vi "MATglobal.vi"(1 "s":bool, 2 "rawdata":T1) -> (0 "rawdata":T1)   [LabVIEW 2009]
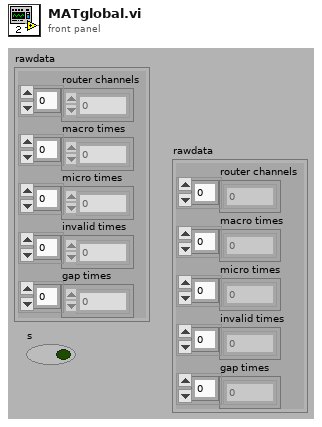
[diagram p1: front panel]
types:
  T1 = cluster{"router channels":u8[], "macro times":u32[], "micro times":u16[], "invalid times":u32[], "gap times":u32[]}
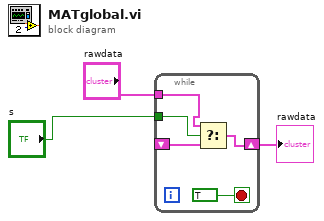
[diagram p0: block diagram]
diagram:
  n1 = while {
    shift-right: [w7] -> w3
    shift-left: _ -> [w8]
    tunnel: "s" -> [w6]
    tunnel: "rawdata" -> [w5]
    stop <- TRUE stop-if-true
    n2 = Select(t=w5, s=w6, f=w8) -> (s? t:f=w7:T1)
  }
  "rawdata" <- w3
